vi "FPGA.vi"() -> ()   [LabVIEW 2016]
uses:
  <vilib>/rvi/Emulation/niFpgaGetClockAttributes.vi
  <vilib>/rvi/Emulation/niFpgaSctlEmulationGetInTimedLoop.vi
  <vilib>/rvi/Emulation/niFpgaEmulationReportErrorSimple.vi
  <vilib>/rvi/eio/common/nirviEmuTemplateMethod_errors.vi
  <vilib>/rvi/Emulation/niFpgaCriticalErrorInLSC.vi
  <vilib>/eio/EIONode/EIONode.xnode
panel:
  in  "Half-period":u32 caption="Count(mSec)"
  in  "Flash":bool
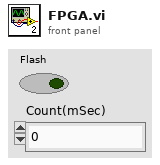
[diagram p1: front panel]
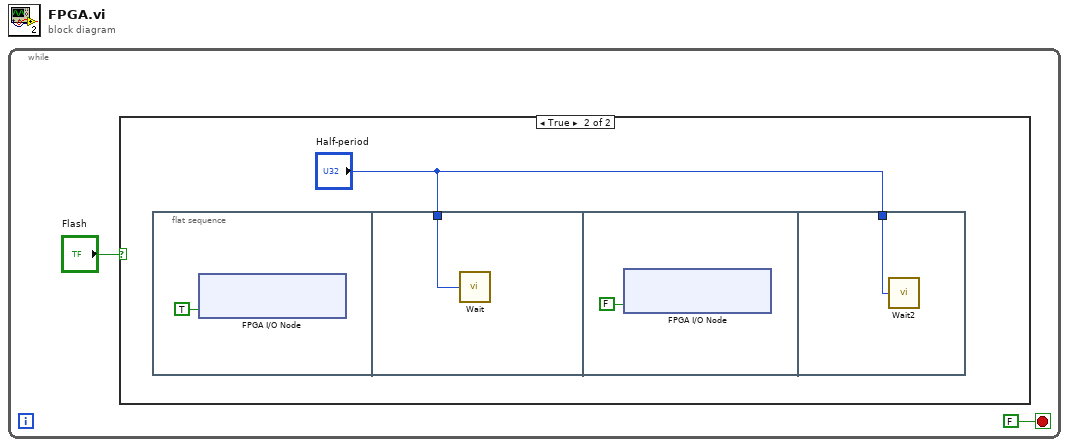
[diagram p0: block diagram]
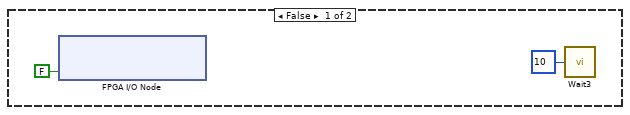
[diagram p2: hidden frame]
diagram:
  n1 = while {
    stop <- FALSE stop-if-true
    n2 = case shown="True" "Flash" {
      frame False {
        n3 = xnode "FPGA I/O Node"("USER FPGA LED"=FALSE) -> ()  [unwired: 1 in, 1 out]
        n4 = call "Wait3"("Count(mSec)"=u32 10) -> ()  [unwired: 1 out]
      }
      frame True {
        n5 = flat-sequence {
          tunnel: "Half-period" -> [w7]
          tunnel: "Half-period" -> [w9]
          frame #0 {
            n6 = xnode "FPGA I/O Node"("USER FPGA LED"=TRUE) -> ()  [unwired: 1 in, 1 out]
          }
          frame #1 {
            n7 = call "Wait"("Count(uSec)"=w7) -> ()  [unwired: 1 out]
          }
          frame #2 {
            n8 = xnode "FPGA I/O Node"("USER FPGA LED"=FALSE) -> ()  [unwired: 1 in, 1 out]
          }
          frame #3 {
            n9 = call "Wait2"("Count(uSec)"=w9) -> ()  [unwired: 1 out]
          }
        }
      }
    }
  }
